vi "Hierarchical VArray to MultiD Array.vi"(8 "error in (no error)":errorcluster, 9 "Element Type":variant, 10 "Hierarchical Array":variant[](array[variant]), 11 "Nulls as Defaults?":bool) -> (0 "error out":errorcluster, 2 "MultiD Array":variant)   [LabVIEW 2020, in "openg_variant.lvlib"]
uses:
  openg_variant.lvlib
  <vilib>/Utility/Data Type/NI_Data Type.lvlib
panel:
  # "EXPERIMENTAL"
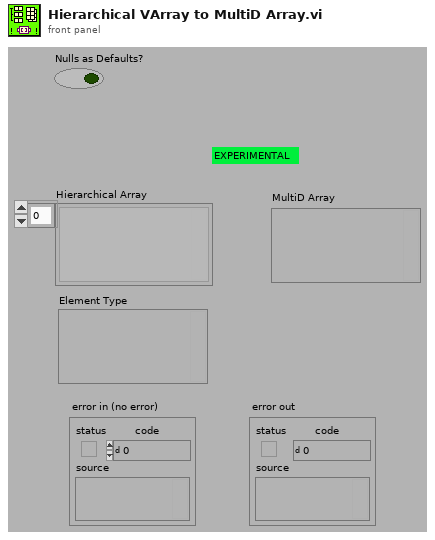
[diagram p1: front panel]
types:
  T1 = typedef "NI_Data Type.lvlib/Data Type.ctl" = enum8{"Invalid Type", "Void", "I8", "I16", "I32", "I64", "U8", "U16", "U32", "U64", "Single Float", "Double Float", "Extended Float", "Single Complex", "Double Complex", "Extended Complex", "Enum U8", "Enum U16", "Enum U32", "Enum U64", "Single Float With Unit", "Double Float With Unit", "Extended Float With Unit", "Single Complex with Unit", "Double Complex with Unit", "Extended Complex with Unit", "Boolean", "String", "Path", "Picture", "Tag", "Array", "Cluster", "Variant", "LV Variant", "Waveform", "Timestamp", "Digital Waveform", "Digital Data", "ExpressData", "Refnum", "External Data", "VI", "Poly VI", "LabVIEW Class Instance", "Fixed Point", "Set Collection", "Map Collection"}
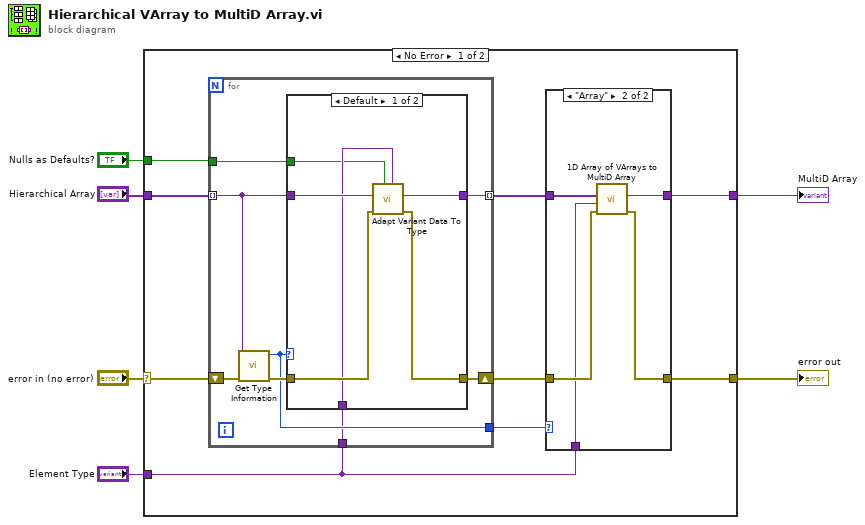
[diagram p0: block diagram]
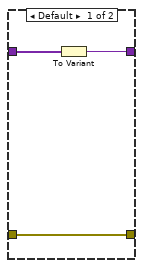
[diagram p2: hidden frame]
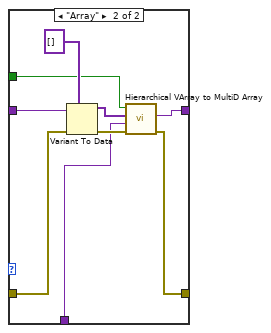
[diagram p3: hidden frame]
diagram:
  n1 = case shown="No Error" "error in (no error)" {
    selector: "error in (no error)" -> [w14 w47]
    tunnel: [w11 w47] -> w6
    tunnel: [w10 _] -> w3
    tunnel: "Hierarchical Array" -> [w15 _]
    tunnel: "Element Type" -> [w8 _]
    tunnel: "Nulls as Defaults?" -> [w7 _]
    frame No Error {
      n2 = for {
        tunnel: w15 -> [w28] mode=indexing
        shift-right: [w30] -> w12
        shift-left: w14 -> [w31]
        tunnel: [w27] -> w13 mode=indexing
        tunnel: [w26] -> w9
        tunnel: w8 -> [w25]
        tunnel: w7 -> [w24]
        n3 = call <vilib>:"Get Type Information.vi"("error in (no error)"=w31, "variant"=w28) -> ("error out"=w29:errorcluster, "type"=w26:T1)  [unwired: 5 in, 3 out]
        n4 = case shown="Default" w26 {
          tunnel: [w34 w41] -> w30
          tunnel: w29 -> [w35 w40]
          tunnel: w28 -> [w37 w46]
          tunnel: [w36 w42] -> w27
          tunnel: w25 -> [w33 w38]
          tunnel: w24 -> [w32 w39]
          frame Default {
            n5 = call "Adapt Variant Data To Type.vi"("Type and Defaults"=w33, "Nulls as Defaults?"=w32, "error in (no error)"=w35, "Variant in"=w37) -> ("error out"=w34:errorcluster, "Variant out"=w36:variant)  [unwired: 6 in]
          }
          frame "Array" {
            n6 = Variant To Data(error in=w40, type=variant[] [], Variant=w46) -> (data=w44:variant[], error out=w43:errorcluster)
            n7 = call "Hierarchical VArray to MultiD Array.vi"("error in (no error)"=w43, "Element Type"=w38, "Hierarchical Array"=w44, "Nulls as Defaults?"=w39) -> ("error out"=w41:errorcluster, "MultiD Array"=w42:variant)  [unwired: 6 in]
          }
        }
      }
      n8 = case shown="\"Array\"" w9 {
        tunnel: w13 -> [w17 w23]
        tunnel: w12 -> [w16 w22]
        tunnel: [w16 w21] -> w11
        tunnel: [w18 w20] -> w10
        tunnel: w8 -> [_ w19]
        frame Default {
          n9 = To Variant(anything=w17) -> (Variant=w18:variant)
        }
        frame "Array" {
          n10 = call "1D Array of VArrays to MultiD Array.vi"("error in (no error)"=w22, "Element Type"=w19, "Array of VArrays"=w23) -> ("error out"=w21:errorcluster, "MultiD Array"=w20:variant)  [unwired: 7 in]
        }
      }
    }
    frame Error {
    }
  }
  "error out" <- w6
  "MultiD Array" <- w3
